vi "Array to Spreadsheet String.vi"() -> ()   [LabVIEW 2018]
doc: "Demonstrates the Array to Spreadsheet String function."
panel:
  out "Resulting Spreadsheet String ('\\' Codes Display)":string
  out "Resulting Spreadsheet String (Normal Display)":string
  in  "Format String":string="%f"
  in  "Delimiter ('\\' Codes Display)":string="\t"
  in  "Original 2D Array":dbl[][](array[numeric])=[[0.0, 1.0, 2.0, 3.0], [4.0, 5.0, 6.0, 7.0], [8.0, 9.0, 10.0, 11.0], [12.0, 13.0, 14.0, 15.0]] format="%#.6g"
  # "Overview: Demonstrates the use of the Array to Spreadsheet String function.\nInstructions:\n1. Run the VI.\n2. Change the Delimiter or Format String and run the VI again to view the results."
  # "You can experiment with these format specifiers or refer to the Format Specifier Syntax in the Help:\n%f - floating-point number with fractional format \n%3d - signed decimal integer with a minimum field width of three characters\n%8.4f - floating-point number, with a minimum field width of eight characters. Four characters correspond to the precision."
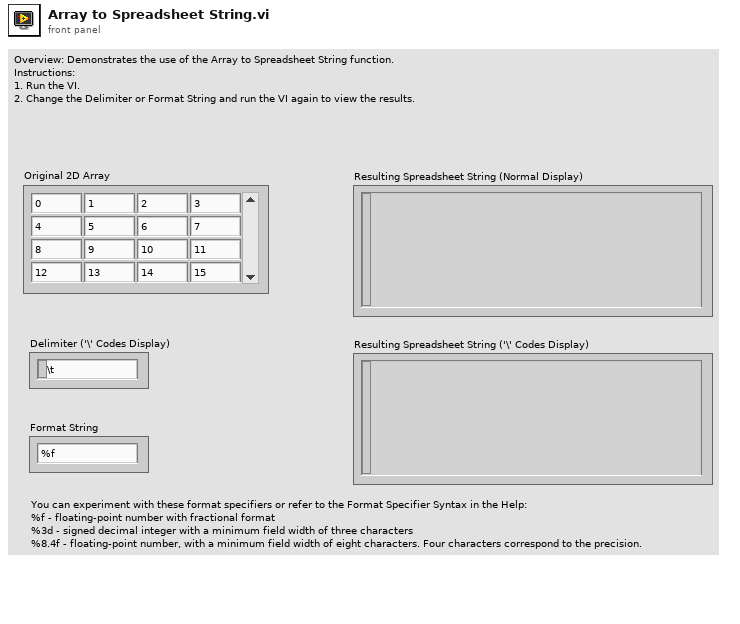
[diagram p1: front panel]
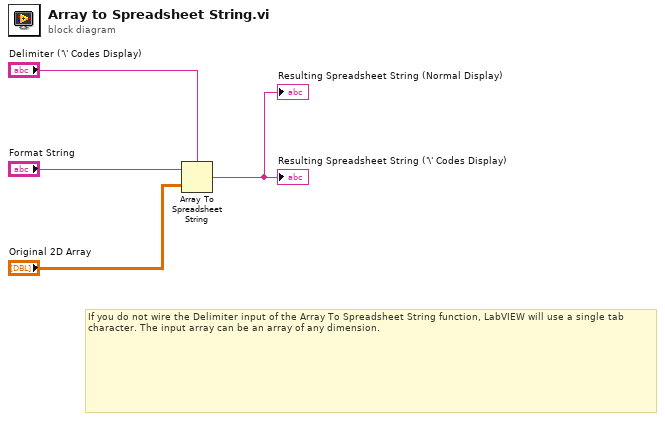
[diagram p0: block diagram]
diagram:
  # "If you do not wire the Delimiter input of the Array To Spreadsheet String function, LabVIEW will use a single tab character. The input array can be an array of any dimension."
  n1 = Array To Spreadsheet String(delimiter (Tab)="Delimiter ('\\' Codes Display)", array="Original 2D Array", 3:"Format String") -> (spreadsheet string=→"Resulting Spreadsheet String (Normal Display)" →"Resulting Spreadsheet String ('\\' Codes Display)":string)
